vi "VIPM_Load File Group Map.vi"(8 "error in (no error)":errorcluster, 10 "File Group Name":string, 11 "Refnum in":T1) -> (0 "error out":errorcluster, 2 "Ordered File Group map":map{string, string[]}(c390), 3 "Refnum out":T1)   [LabVIEW 2019]
doc: "Load all vi, vims, ctl and lvclass paths and order them in a map by the first folder name. \nThe file name is removed."
uses:
  <vilib>/Utility/config.llb/NI_LVConfig.lvlib
  <vilib>/Utility/config.llb/Config Data RefNum.ctl
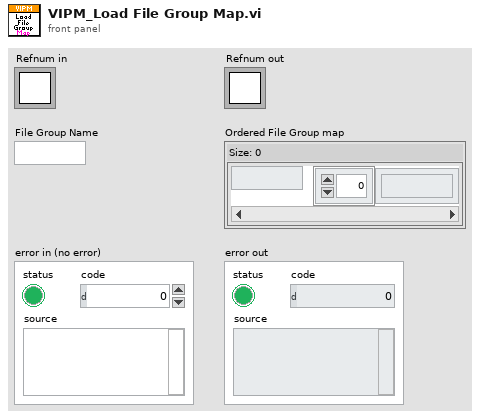
[diagram p1: front panel]
types:
  T1 = typedef "NI_LVConfig.lvlib/Config Data RefNum.ctl" = refnum<k1>
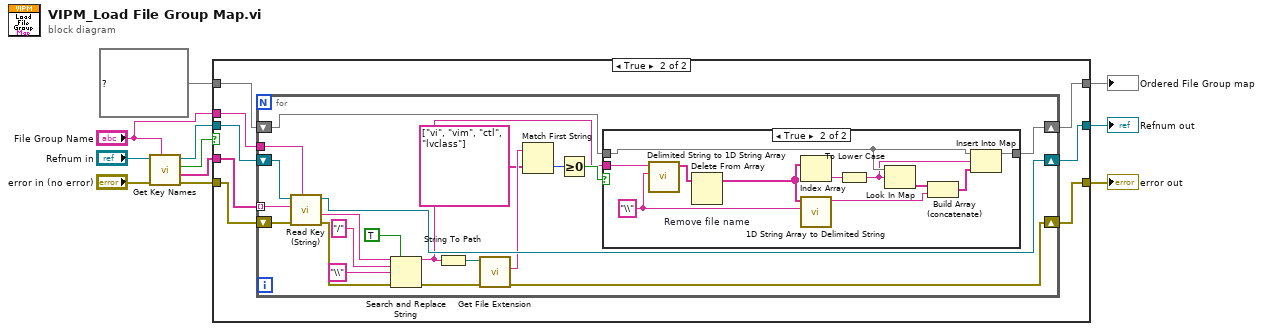
[diagram p0: block diagram]
diagram:
  n1 = call <vilib>:"Get Key Names.vi"("section"="File Group Name", "error in (no error)"="error in (no error)", "refnum"="Refnum in") -> ("error out"=w7:errorcluster, "key names"=w8:string[], "section exists?"=w3:bool, "refnum out"=w5:T1)  [unwired: 5 in]
  n2 = case shown="True" w3 {
    tunnel: [w14 w17] -> w4
    tunnel: w5 -> [w14 w22]
    tunnel: [w13 w18] -> w6
    tunnel: w7 -> [w13 w19]
    tunnel: w8 -> [_ w21]
    tunnel: "File Group Name" -> [_ w20]
    tunnel: [w12 w16] -> w10
    tunnel: map{string, string[]} {} ("map") -> [w12 w15]
    frame False {
    }
    frame True {
      n3 = for {
        tunnel: w21 -> [w41] mode=indexing
        tunnel: w20 -> [w40]
        shift-right: [w39] -> w17
        shift-left: w22 -> [w42]
        shift-right: [w33] -> w18
        shift-left: w19 -> [w38]
        shift-right: [w24] -> w16
        shift-left: w15 -> [w23]
        n4 = call <vilib>:"Read Key (String).vi"("section"=w40, "error in (no error)"=w38, "key"=w41, "refnum"=w42) -> ("error out"=w37:errorcluster, "value"=w30:string, "refnum out"=w39:T1)  [unwired: 4 in, 1 out]
        n5 = Search and Replace String(replace all?=TRUE ("replace all? (F)"), input string=w30, search string="/", replace string="\\" ("search string"), error in=w37) -> (result string=w25:string, error out=w31:errorcluster)  [unwired: 3 in, 2 out]
        n6 = String To Path(string=w25) -> (path=w32:path)
        n7 = call <vilib>:"Get File Extension.vi"("error in (no error)"=w31, "file"=w32) -> ("error out"=w33:errorcluster, "lowercase file extension"=w35:string)  [unwired: 5 in, 3 out]
        n8 = Match First String(2:string[] ["vi", "vim", "ctl", "lvclass"] ("string array"), 3:w35) -> (0:w36:i32)  [unwired: 1 out]
        n9 = Greater Or Equal To 0?(x=w36) -> (x >= 0?=w26:bool)
        n10 = case shown="True" w26 {
          tunnel: w25 -> [_ w54]
          tunnel: [w43 w48] -> w24
          tunnel: w23 -> [w43 w50]
          frame False {
          }
          frame True {
            w52 = "\\" ("search string")
            n11 = call <vilib>:"Delimited String to 1D String Array.vi"("delimiter"=w52, "delimited string"=w54) -> ("string array"=w53:string[])  [unwired: 9 in]
            n12 = Delete From Array "Remove file name"(array=w53) -> (array with subset deleted=w51:string[])  [unwired: 2 in, 1 out]
            n13 = Index Array(array=w51) -> (element=w49:string)  [unwired: 1 in]
            n14 = call <vilib>:"1D String Array to Delimited String.vi"("delimiter"=w52, "string array"=w51) -> ("delimited string"=w45:string)  [unwired: 9 in]
            n15 = To Lower Case(string=w49) -> (all lower case string=w47:string)
            n16 = Look In Map(map=w50, key=w47) -> (value=w46:string[])  [unwired: 1 in, 1 out]
            n17 = Build Array (concatenate)(w46, w45) -> (w44:string[])
            n18 = Insert Into Map(map in=w50, key=w47, value=w44) -> (map out=w48:map{string, string[]})  [unwired: 2 out]
          }
        }
      }
    }
  }
  "Ordered File Group map" <- w10
  "error out" <- w6
  "Refnum out" <- w4
